vi "Remote Shutdown Status.vi"() -> (2 "Subsystem Status":T1)   [LabVIEW 2014]
uses:
  Vehicle Status/Subsystem Status.ctl
  Global Data.vi
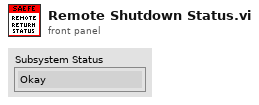
[diagram p1: front panel]
types:
  T1 = typedef "Subsystem Status.ctl" = enum16{"Okay", "Short Warning", "Long Warning", "Return to Pits", "Error", "Danger"}
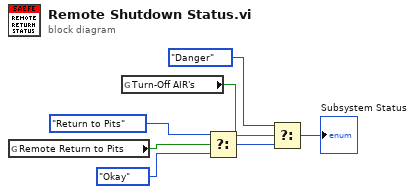
[diagram p0: block diagram]
diagram:
  n1 = global read "Global Data.vi" "Remote Return to Pits"() -> (w6:bool)
  n2 = global read "Global Data.vi" "Turn-Off AIR's"() -> (w2:bool)
  n3 = Select(t=Subsystem_Status."Return to Pits", s=w6, f=Subsystem_Status."Okay" ("Subsystem Status")) -> (s? t:f=w4:T1)
  n4 = Select(t=Subsystem_Status."Danger", s=w2, f=w4) -> (s? t:f=→"Subsystem Status":T1)
